vi "test harness_FXP_X_minus_Nx_times_ye_singleAxis.vi"(8 "error in (no error)":errorcluster, 11 "TestCase in":refnum<class "FXP_observer_TestCase.lvclass">) -> (0 "error out":errorcluster, 3 "TestCase out":refnum<class "FXP_observer_TestCase.lvclass">)   [LabVIEW 2017, in "FXP_observer_TestCase.lvclass"]
uses:
  FXP_observer_TestCase.lvclass
  <vilib>/rvi/DesktopExecutionNode/Execution/niFpgaDEN_Execute.vi
  <vilib>/rvi/DesktopExecutionNode/DesktopExecutionNode.xnode
  <vilib>/addons/_JKI Toolkits/VI Tester/TestCase.llb/TestCase.lvclass
  C:/Program Files (x86)/National Instruments/LabVIEW 2017/vi.lib/addons/_JKI Toolkits/VI Tester/TestCase.llb/TestCase.lvclass
panel:
  out "error (x_uk)":errorcluster
  out "xerr (expected)":fxp<+/-,64,11>[](array[numeric])
  out "xer":fxp<+/-,32,5>[](array[numeric])
  in  "xk_1_2_mem":fxp<+/-,32,5>[](array[numeric])=[2.0, 4.0, 3.0, 6.0, 0.25, 0.0, 0.0, 0.0, 0.0, 0.0, 0.0, 0.0, 0.0, 0.0, 0.0, 0.0, 0.0, 0.0, 0.0, 0.0, 0.0, 0.0, 0.0, 0.0, 0.0, 0.0, 0.0, 0.0, 0.0, 0.0, 0.0, 0.0, 0.0, 0.0, 0.0, 0.0, 0.0, 0.0, 0.0, 0.0, 0.0, 0.0, 0.0, 0.0, 0.0, 0.0, 0.0, 0.0, 0.0, 0.0]
  in  "Nx":fxp<+/-,32,5>[](array[numeric])=[0.20000000298023224, 0.29999999701976776, 0.3999999985098839, 1.2999999970197678, 1.2000000029802322, 0.0, 0.0, 0.0, 0.0, 0.0, 0.0, 0.0, 0.0, 0.0, 0.0, 0.0, 0.0, 0.0, 0.0, 0.0, 0.0, 0.0, 0.0, 0.0, 0.0, 0.0, 0.0, 0.0, 0.0, 0.0, 0.0, 0.0, 0.0, 0.0, 0.0, 0.0, 0.0, 0.0, 0.0, 0.0, 0.0, 0.0, 0.0, 0.0, 0.0, 0.0, 0.0, 0.0, 0.0, 0.0]
  in  "ref(k)_x":fxp<+/-,32,5>=2.0
  in  "yd_est_x":fxp<+/-,32,5>=0.25
  in  "NS":u8=5
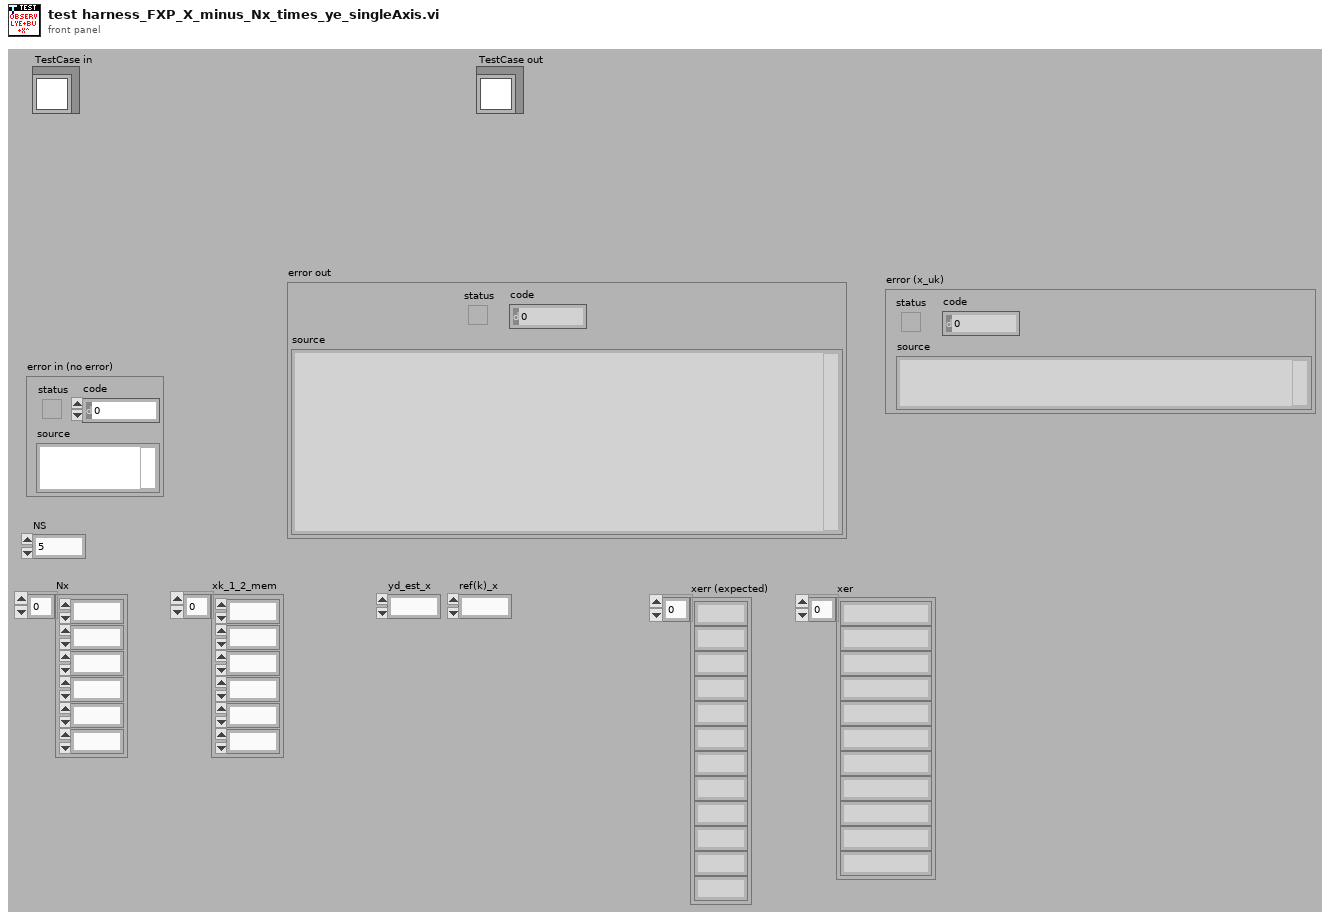
[diagram p1: front panel]
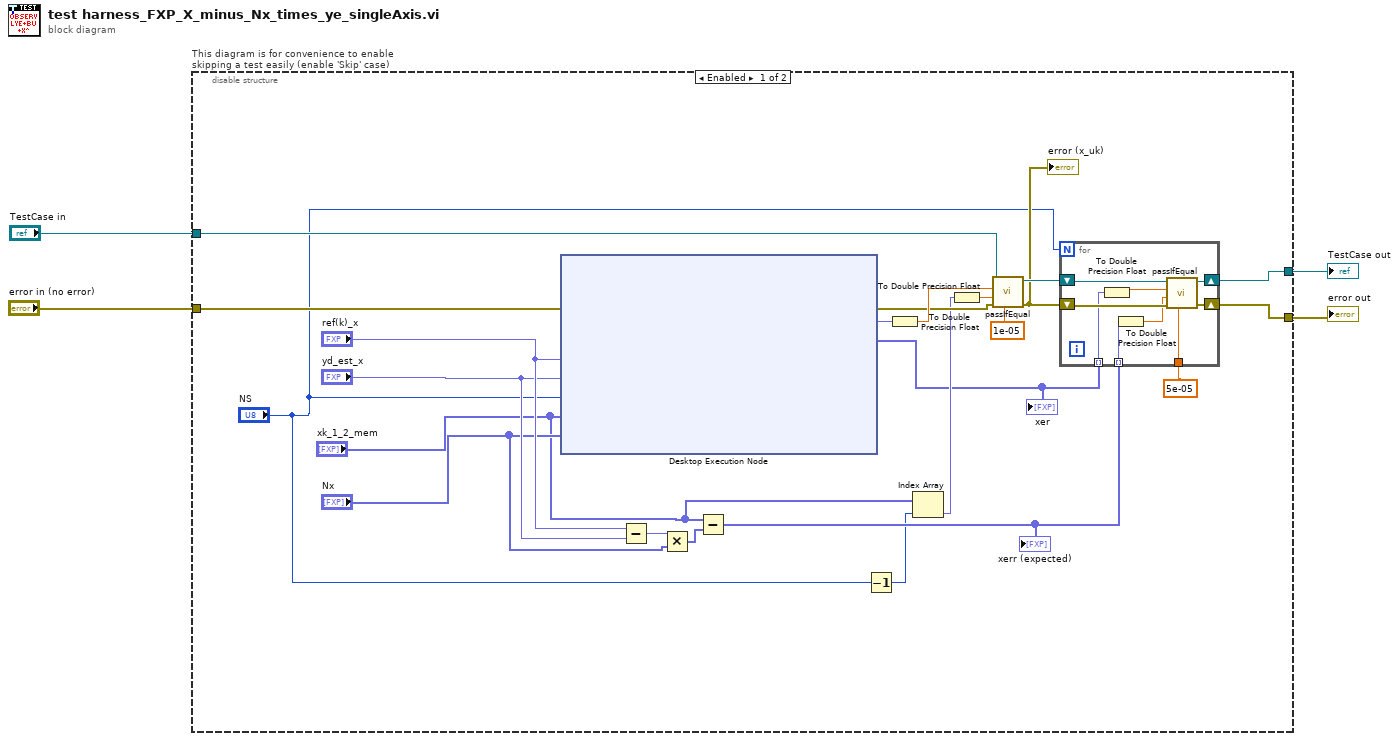
[diagram p0: block diagram]
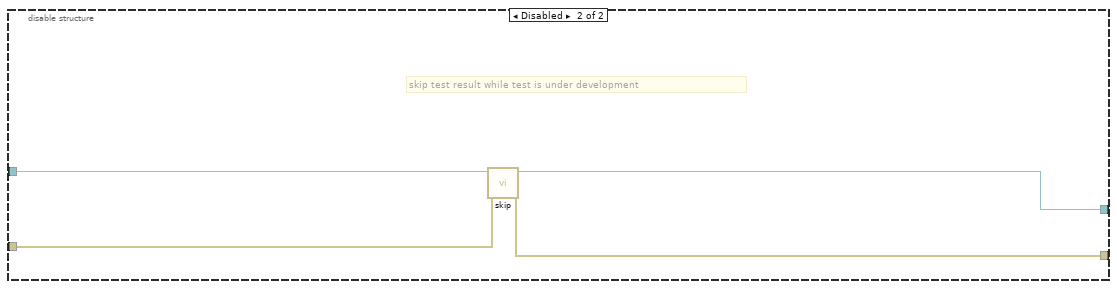
[diagram p2: hidden frame]
diagram:
  n1 = disable-structure "This diagram is for convenience to enable skipping a test easily (enable 'Skip' case)" shown="Enabled" {
    disable-tunnel: "TestCase in" -> [w27 w40]
    disable-tunnel: [w10 w38] -> w1
    disable-tunnel: [w9 w39] -> w3
    disable-tunnel: "error in (no error)" -> [w23 w37]
    frame Enabled {
      n2 = xnode "Desktop Execution Node"("Error In"=w23, "ref(k)_x"="ref(k)_x", "yd_est_x"="yd_est_x", "NS + 1"="NS", "xk_1_2_mem"="xk_1_2_mem", "Nx"="Nx") -> ("Error Out"=w24:errorcluster, "xu_k"=w14:fxp<+/-,32,5>, "xerr"=w5:fxp<+/-,18,5>[])
      "xer" <- w5
      n3 = Subtract(x="ref(k)_x", y="yd_est_x") -> (x-y=w17:fxp<+/-,33,6>)
      n4 = Multiply(x=w17, y="Nx") -> (x*y=w15:fxp<+/-,64,10>[])
      n5 = Subtract(x="xk_1_2_mem", y=w15) -> (x-y=w11:fxp<+/-,64,11>[])
      "xerr (expected)" <- w11
      n6 = Decrement(x="NS") -> (x-1=w8:u8)
      n7 = To Double Precision Float(number=w14) -> (double precision float=w25:dbl)
      n8 = Index Array(array="xk_1_2_mem", index=w8) -> (element=w21:fxp<+/-,32,5>)
      n9 = To Double Precision Float(number=w21) -> (double precision float=w22:dbl)
      n10 = call-dynamic "passIfEqual.vi"("delta (optional)"=1e-05 ("del u_x"), "error in (no error)"=w24, "y"=w22, "x"=w25, "TestCase in"=w27) -> ("error out"=w12:errorcluster, "TestCase out"=w13:refnum<class "FXP_observer_TestCase.lvclass">)  [unwired: 5 in]
      "error (x_uk)" <- w12
      n11 = for {
        N: "NS" -> [_]
        shift-right: [w36] -> w10
        shift-left: w13 -> [w33]
        shift-right: [w35] -> w9
        shift-left: w12 -> [w34]
        tunnel: w11 -> [w32] mode=indexing
        tunnel: 5e-05 ("del u_x") -> [w29]
        tunnel: w5 -> [w28] mode=indexing
        n12 = To Double Precision Float(number=w28) -> (double precision float=w30:dbl)
        n13 = To Double Precision Float(number=w32) -> (double precision float=w31:dbl)
        n14 = call-dynamic "passIfEqual.vi"("delta (optional)"=w29, "error in (no error)"=w34, "y"=w31, "x"=w30, "TestCase in"=w33) -> ("error out"=w35:errorcluster, "TestCase out"=w36:refnum<class "FXP_observer_TestCase.lvclass">)  [unwired: 5 in]
      }
    }
    frame Disabled {
      # "skip test result while test is under development"
      n15 = call <vilib>:"skip.vi"("error in (no error)"=w37, "TestCase in"=w40) -> ("error out"=w39:errorcluster, "TestCase out"=w38:refnum<class "FXP_observer_TestCase.lvclass">)  [unwired: 8 in]
    }
  }
  "error out" <- w3
  "TestCase out" <- w1
